vi "etlUSBSetMode.vi"(1 "lens":enum16{"0", "1"}(ring), 2 "mode":u16(ring) items=["controlled"]) -> ()   [LabVIEW 2017]
uses:
  globalDevices.vi
panel:
  out "concatenated string":string
  out "read buffer":string
  out "return count":u32
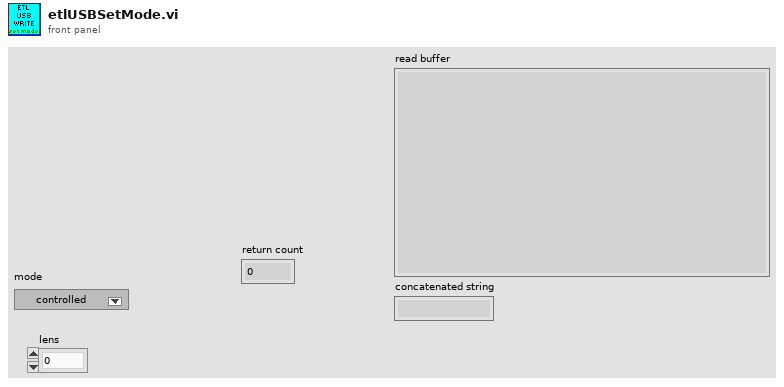
[diagram p1: front panel]
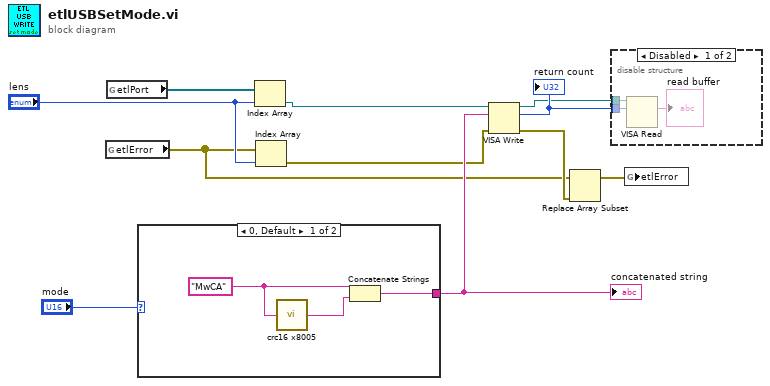
[diagram p0: block diagram]
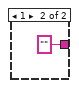
[diagram p3: hidden frame]
diagram:
  n1 = global read "globalDevices.vi" "etlError"() -> (w3:errorcluster[])
  n2 = global read "globalDevices.vi" "etlPort"() -> (w7:refnum<visa-resource-name>[])
  n3 = case shown="0, Default" "mode" {
    tunnel: [w12 ""] -> w10
    frame 0, Default {
      w13 = "MwCA"
      n4 = call "crc16 x8005.vi"("message"=w13) -> ("CRC16"=w14:string)  [unwired: 4 in]
      n5 = Concatenate Strings(w13, w14) -> (w12:string)
    }
    frame 1 {
    }
  }
  "concatenated string" <- w10
  n6 = Index Array(array=w7, index="lens") -> (element=w5:refnum<visa-resource-name>)
  n7 = Index Array(array=w3, index="lens") -> (element=w4:errorcluster)
  n8 = VISA Write(VISA resource name=w5, write buffer=w10, error in (no error)=w4) -> (VISA resource name out=w1:refnum<visa-resource-name>, return count=w2:u32, error out=w9:errorcluster)
  "return count" <- w2
  n9 = Replace Array Subset(array=w3, new element=w9) -> (w8:errorcluster[])  [unwired: 1 in]
  n10 = disable-structure shown="Disabled" {
    disable-tunnel: w2 -> [w18 _]
    disable-tunnel: w1 -> [w17 _]
    frame Disabled {
      n11 = VISA Read(VISA resource name=w17, byte count=w18) -> (read buffer=→"read buffer":string)  [unwired: 1 in, 3 out]
    }
    frame Enabled {
    }
  }
  n12 = global write "globalDevices.vi" "etlError"(w8) -> ()
